vi "GetPumpData.vi"(7 "LabVIEW Web Service Request":refnum<class "Web Request.lvclass">) -> ()   [LabVIEW 2019]
uses:
  <vilib>/wsapi/Web Request.lvclass
  Controls/RPi HMI Mode.ctl
  Controls/Pump Data.ctl
  Controls/HMI Header.ctl
  Controls/Tank CMDs.ctl
  Controls/HMI Tog Buttons.ctl
  Controls/HMI Mom Buttons.ctl
panel:
  # "Use the Web Service Request input terminal to call the VIs on the Web Services palette. Do not remove it from the connector pane unless you don't need access to the palette."
  # "Each additional control wired to the connector pane will be available as an input in the URL. To include an indicator in terminal-mode output (the default setting), it must also be wired to the connector pane."
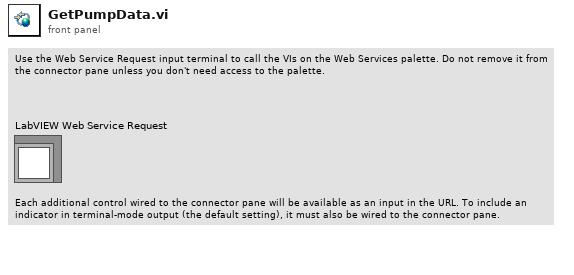
[diagram p1: front panel]
types:
  T1 = typedef "Pump Data.ctl" = cluster{"Voltages":dbl[], "PumpCurrent":dbl[], "Speed":dbl[], "ControllerCurrent":dbl[], "Pressure":dbl[], "Flow":dbl[], "Elapsed Time (Display)":dbl[], "Avg Pressure":dbl, "Avg Speed":dbl, "Elapsed Time":dbl[]}
  T2 = typedef "HMI Header.ctl" = cluster{"Line 1":string, "Line 2":string, "Line 3":string, "Line 4":string}
  T3 = typedef "Tank CMDs.ctl" = cluster{"PS CMD":dbl, "Press CMD":dbl, "Temp 1 CMD":dbl, "Temp 2 CMD":dbl}
  T4 = typedef "HMI Tog Buttons.ctl" = cluster{"Start Test":bool, "Toggle Spare 1":bool, "Toggle Spare 2":bool, "Toggle Spare 3":bool, "Toggle Spare 4":bool, "Toggle Spare 5":bool}
  T5 = typedef "HMI Mom Buttons.ctl" = cluster{"Stop":bool, "Reset Timers":bool, "Log Fuel Change":bool, "Alarm Dismiss":bool}
  T6 = cluster{"Error":errorcluster, "Pump Data":T1, "Tank Data":cluster{"PS Actual (V):":dbl, "Temp1":dbl, "Temp2":dbl}, "Power Relays":cluster{"Pump 1":bool, "Pump 2":bool, "Pump 3":bool, "Pump 4":bool, "Pump 5":bool, "Pump 6":bool}, "Pump CMDs":dbl[], "HMI Header":T2, "Tank CMDs":T3, "HMI Tog Buttons":T4, "In Test":bool, "HMI Command":bool, "HMI Mom Buttons":T5, "Controller Config":cluster{"CommSeg":i32, "PWM?":bool, "Frequency":i32, "Low Command":dbl, "High Command":dbl, "Stop Command":dbl, "Command Step":dbl, "Solenoid Stop?":bool, "Controller?":bool, "Invert PWM":bool}, "Alarm":bool, "Alarm Message 1":string, "Alarm Message 2":string, "Recording":bool, "Serial Numbers":string[], "Pumps Present":bool[], "CPU Usage":dbl}
  T7 = cluster{"CommSeg":i32, "PWM?":bool, "Frequency":i32, "Low Command":dbl, "High Command":dbl, "Stop Command":dbl, "Command Step":dbl, "Solenoid Stop?":bool, "Controller?":bool, "Invert PWM":bool}
  T8 = typedef "RPi HMI Mode.ctl" = enum16{"Init", "Write Data", "Read from RPi", "Write to RPi", "Read HMI Cluster"}
  T9 = typedef "HMI Cluster.ctl" = cluster{"Error":errorcluster, "COM Ref":refnum<visa-resource-name>, "Pump Data":T1, "Tank Data":cluster{"PS Actual (V):":dbl, "Temp1":dbl, "Temp2":dbl}, "Power Relays":cluster{"Pump 1":bool, "Pump 2":bool, "Pump 3":bool, "Pump 4":bool, "Pump 5":bool, "Pump 6":bool}, "Pump CMDs":dbl[], "HMI Header":T2, "Tank CMDs":T3, "HMI Tog Buttons":T4, "In Test":bool, "HMI Command":bool, "HMI Mom Buttons":T5, "Controller Config":T10, "Alarm":bool, "Alarm Message 1":string, "Alarm Message 2":string, "Recording":bool, "Serial Numbers":string[], "Pumps Present":bool[]}
  T10 = typedef "Controller Config.ctl" = cluster{"Controller Name":T11, "CommSeg":i32, "PWM?":bool, "Frequency":i32, "Low Command":dbl, "High Command":dbl, "Stop Command":dbl, "Command Step":dbl, "Solenoid Stop?":bool, "Controller?":bool, "Invert PWM":bool}
  T11 = typedef "Controller Names.ctl" = enum16{"Kuhnke", "Helbako BLDC", "Conti", "Hella BLDC OL PWM", "Hella BLDC Turbine OL PWM", "Hella BLDC Pressure", "Helbako (old)", "TI PWM", "PSA", "Hella Gas", "Hella Diesel", "8 Comm", "10 Comm", "8 Comm Hella", "10 Comm Hella", "8 Comm Omron", "10 Comm Omron", "8 Comm Nissan", "10 Comm Nissan"}
  T12 = cluster{"PS Actual (V):":dbl, "Temp1":dbl, "Temp2":dbl}
  T13 = cluster{"Pump 1":bool, "Pump 2":bool, "Pump 3":bool, "Pump 4":bool, "Pump 5":bool, "Pump 6":bool}
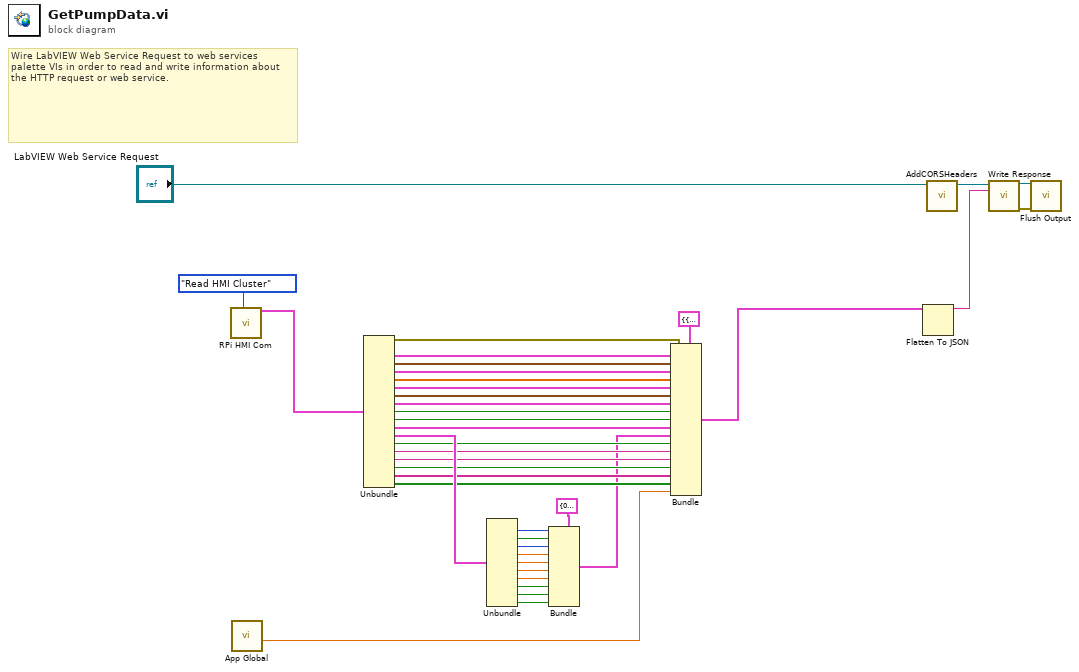
[diagram p0: block diagram]
diagram:
  # "Wire LabVIEW Web Service Request to web services palette VIs in order to read and write information about the HTTP request or web service."
  n1 = call "RPi HMI Com.vi"("RPi HMI Mode"=RPi_HMI_Mode."Read HMI Cluster") -> ("HMI Cluster"=w37:T9)  [unwired: 18 in]
  n2 = call "App Global.vi"() -> ("CPU Usage OUT"=w5:dbl)  [unwired: 9 in, 2 out]
  n3 = Unbundle(w37) -> ("Error"=w34:errorcluster, "Pump Data"=w33:T1, "Tank Data"=w32:T12, "Power Relays"=w31:T13, "Pump CMDs"=w30:dbl[], "HMI Header"=w29:T2, "Tank CMDs"=w28:T3, "HMI Tog Buttons"=w27:T4, "In Test"=w26:bool, "HMI Command"=w25:bool, "HMI Mom Buttons"=w24:T5, "Controller Config"=w36:T10, "Alarm"=w23:bool, "Alarm Message 1"=w22:string, "Alarm Message 2"=w21:string, "Recording"=w20:bool, "Serial Numbers"=w19:string[], "Pumps Present"=w18:bool[])  [unwired: 1 out]
  n4 = Unbundle(w36) -> ("CommSeg"=w16:i32, "PWM?"=w15:bool, "Frequency"=w14:i32, "Low Command"=w13:dbl, "High Command"=w12:dbl, "Stop Command"=w11:dbl, "Command Step"=w10:dbl, "Solenoid Stop?"=w9:bool, "Controller?"=w8:bool, "Invert PWM"=w7:bool)  [unwired: 1 out]
  n5 = Bundle(cluster=T7 {"CommSeg"=0, "PWM?"=FALSE, "Frequency"=0, "Low Command"=0.0, "High Command"=0.0, "Stop Command"=0.0, "Command Step"=0.0, "Solenoid Stop?"=FALSE, "Controller?"=FALSE, "Invert PWM"=FALSE} ("Controller Config"), "CommSeg"=w16, "PWM?"=w15, "Frequency"=w14, "Low Command"=w13, "High Command"=w12, "Stop Command"=w11, "Command Step"=w10, "Solenoid Stop?"=w9, "Controller?"=w8, "Invert PWM"=w7) -> (w6:T7)
  n6 = Bundle(cluster=T6 {"Error"={"status"=FALSE, "code"=0, "source"=""}, "Pump Data"={"Voltages"=[], "PumpCurrent"=[], "Speed"=[], "ControllerCurrent"=[], "Pressure"=[], "Flow"=[], "Elapsed Time (Display)"=[], "Avg Pressure"=0.0, "Avg Speed"=0.0, "Elapsed Time"=[4074.9003000000002, 4074.9003000000002, 4074.9003000000002, 4074.9003000000002, 4074.9003000000002, 4074.9003000000002]}, "Tank Data"={"PS Actual (V):"=0.0, "Temp1"=0.0, "Temp2"=0.0}, "Power Relays"={"Pump 1"=FALSE, "Pump 2"=FALSE, "Pump 3"=FALSE, "Pump 4"=FALSE, "Pump 5"=FALSE, "Pump 6"=FALSE}, "Pump CMDs"=[], "HMI Header"={"Line 1"="", "Line 2"="", "Line 3"="", "Line 4"=""}, "Tank CMDs"={"PS CMD"=0.0, "Press CMD"=0.0, "Temp 1 CMD"=0.0, "Temp 2 CMD"=0.0}, "HMI Tog Buttons"={"Start Test"=FALSE, "Toggle Spare 1"=FALSE, "Toggle Spare 2"=FALSE, "Toggle Spare 3"=FALSE, "Toggle Spare 4"=FALSE, "Toggle Spare 5"=FALSE}, "In Test"=FALSE, "HMI Command"=FALSE, "HMI Mom Buttons"={"Stop"=FALSE, "Reset Timers"=FALSE, "Log Fuel Change"=FALSE, "Alarm Dismiss"=FALSE}, "Controller Config"={"CommSeg"=0, "PWM?"=FALSE, "Frequency"=0, "Low Command"=0.0, "High Command"=0.0, "Stop Command"=0.0, "Command Step"=0.0, "Solenoid Stop?"=FALSE, "Controller?"=FALSE, "Invert PWM"=FALSE}, "Alarm"=FALSE, "Alarm Message 1"="", "Alarm Message 2"="", "Recording"=FALSE, "Serial Numbers"=[], "Pumps Present"=[], "CPU Usage"=0.0} ("HMI Cluster"), "Error"=w34, "Pump Data"=w33, "Tank Data"=w32, "Power Relays"=w31, "Pump CMDs"=w30, "HMI Header"=w29, "Tank CMDs"=w28, "HMI Tog Buttons"=w27, "In Test"=w26, "HMI Command"=w25, "HMI Mom Buttons"=w24, "Controller Config"=w6, "Alarm"=w23, "Alarm Message 1"=w22, "Alarm Message 2"=w21, "Recording"=w20, "Serial Numbers"=w19, "Pumps Present"=w18, "CPU Usage"=w5) -> (w39:T6)
  n7 = Flatten To JSON(anything=w39) -> (JSON string=w1:string)  [unwired: 2 in, 1 out]
  n8 = call "AddCORSHeaders.vi"("Web Request in"="LabVIEW Web Service Request") -> ("Web Request out"=w2:refnum<class "Web Request.lvclass">)  [unwired: 10 in]
  n9 = call <vilib>:"Write Response.vi"("LabVIEW Web Service Request"=w2, "response string"=w1) -> ("LabVIEW Web Service Request out"=w3:refnum<class "Web Request.lvclass">, "error out"=w4:errorcluster)  [unwired: 12 in]
  n10 = call <vilib>:"Flush Output.vi"("LabVIEW Web Service Request"=w3, "error in (no error)"=w4) -> ()  [unwired: 12 in, 2 out]
